vi "SiosIfmDLLVersionString.vi"() -> (0 "DLL Version":string)   [LabVIEW 2009]
uses:
  siosifm.dll
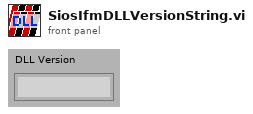
[diagram p1: front panel]
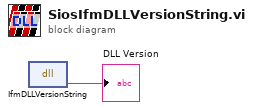
[diagram p0: block diagram]
diagram:
  n1 = dll-call lib="C:/WORK/Artem/RE-10/SIOS_IfmDLL/siosifm.dll" fn="IfmDLLVersionString"() -> ("DLL_Version"=→"DLL Version":string)  [unwired: 3 in, 2 out]
